vi "MU Save Register Ex.vi"(6 "values":u32[](array[numeric]), 7 "registerCount":u32, 8 "error in (no error)":errorcluster, 9 "registerAddress":u32, 10 "filepath":string, 11 "handle":u64) -> (0 "error out (no error)":errorcluster, 3 "function return":u32)   [LabVIEW 2017, in "MU_3SL_interface.lvlib"]
uses:
  MU_3SL_interface.lvlib
  lib/MU_3SL_interface.dll
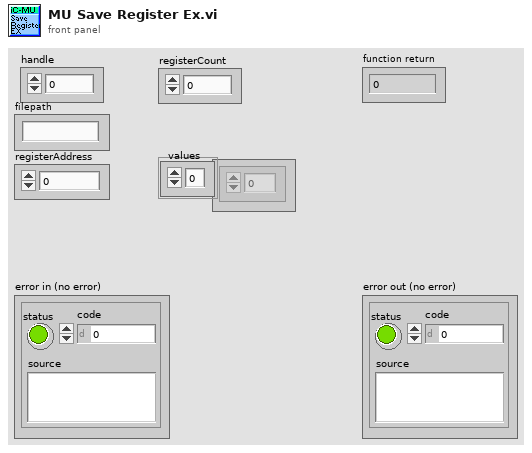
[diagram p1: front panel]
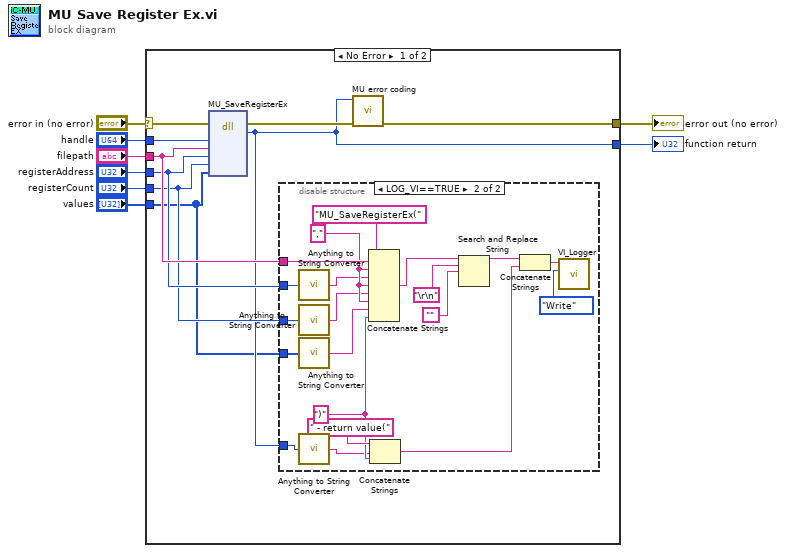
[diagram p0: block diagram]
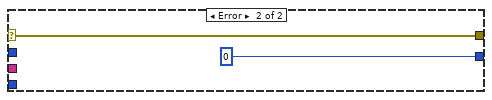
[diagram p3: hidden frame]
diagram:
  n1 = case shown="No Error" "error in (no error)" {
    selector: "error in (no error)" -> [w14 w39]
    tunnel: [w10 u32 0 ("return type")] -> w8
    tunnel: "handle" -> [w17 _]
    tunnel: "filepath" -> [w13 _]
    tunnel: "registerAddress" -> [w12 _]
    tunnel: "registerCount" -> [w11 _]
    tunnel: [w15 w39] -> w3
    tunnel: "values" -> [w9 _]
    frame No Error {
      n2 = dll-call lib="C:/Users/bes/AppData/Roaming/work/mu_9so/icsubmodules/soft_mu_3sl_master/lv_interface/lib/MU_3SL_interface**.*" fn="MU_SaveRegisterEx"(error in=w14, "handle"=w17, "filepath"=w13, "registerAddress"=w12, "registerCount"=w11, "values"=w9) -> (error out=w16:errorcluster, "return type"=w10:u32)  [unwired: 7 in, 1 out]
      n3 = disable-structure shown="LOG_VI==TRUE" {
        disable-tunnel: w10 -> [_ w19]
        disable-tunnel: w12 -> [_ w25]
        disable-tunnel: w11 -> [_ w23]
        disable-tunnel: w13 -> [_ w32]
        disable-tunnel: w9 -> [_ w21]
        frame condition #0 {
        }
        frame condition #1 (active) {
          w30 = ")" ("string")
          w31 = "," ("string")
          n4 = call "Anything to String Converter.vi"("anything"=w25) -> ("String"=w24:string)
          n5 = call "Anything to String Converter.vi"("anything"=w23) -> ("String"=w22:string)
          n6 = call "Anything to String Converter.vi"("anything"=w21) -> ("String"=w20:string)
          n7 = call "Anything to String Converter.vi"("anything"=w19) -> ("String"=w18:string)
          n8 = Concatenate Strings("MU_SaveRegisterEx(" ("Info in"), w32, w31, w24, w31, w22, w31, w20, w30) -> (w27:string)
          n9 = Concatenate Strings(" - return value(" ("string"), w18, w30) -> (w35:string)
          n10 = Search and Replace String(input string=w27, search string="\r\n", replace string="") -> (result string=w26:string)  [unwired: 5 in, 3 out]
          n11 = Concatenate Strings(w26, w35) -> (w34:string)
          n12 = call "VI_Logger.vi"("Action (Read)"=enum16{"Write", "Read"}."Write", "Info in"=w34) -> ()  [unwired: 8 in, 2 out]
        }
      }
      n13 = call "MU error coding.vi"("error in (no error)"=w16, "function return in"=w10) -> ("error out"=w15:errorcluster)  [unwired: 9 in]
    }
    frame Error {
    }
  }
  "function return" <- w8
  "error out (no error)" <- w3
